vi "Error.vi"(6 "Station":T1(ring), 7 "timeout ms (-1)":i32=-1, 8 "error out":errorcluster, 9 "VI Name":string, 10 "error":errorcluster, 11 "Socket":i32) -> (0 "error out 2":errorcluster)   [LabVIEW 2019, in "Unit Test Engine Tools.lvlib"]
uses:
  Unit Test Engine Tools.lvlib
  LVUT Global 1.vi
  <resource>/objmgr/ni.dex.rc
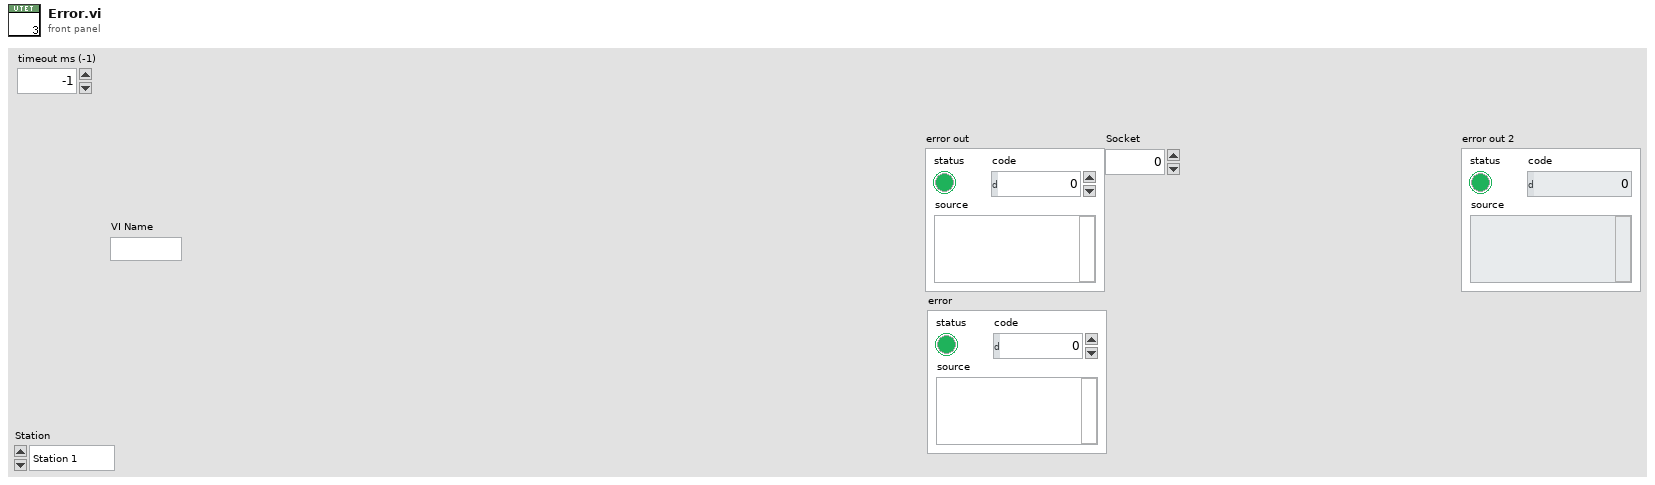
[diagram p1: front panel]
types:
  T1 = enum16{"Station 1", "Station 2", "Station 3", "Station 4"}
  T2 = cluster{"Socket":i32, "error in":errorcluster, "VI Name":string}
  T3 = cluster{"Socket":i32, "error IO":errorcluster, "VI Name":string}
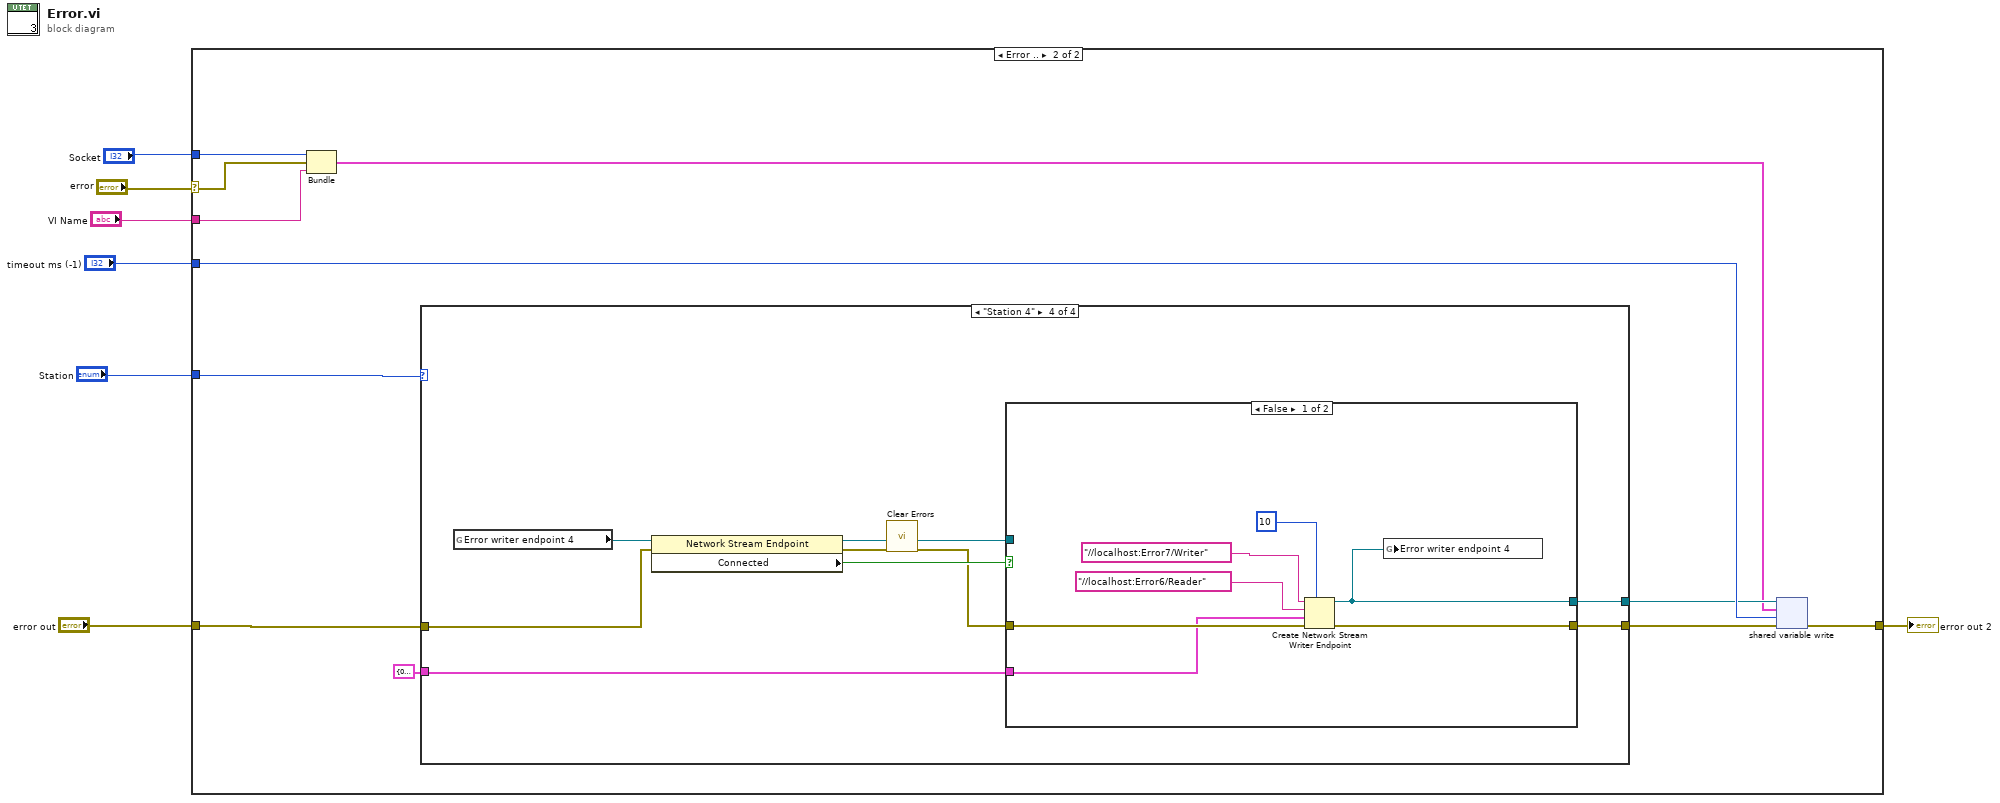
[diagram p0: block diagram]
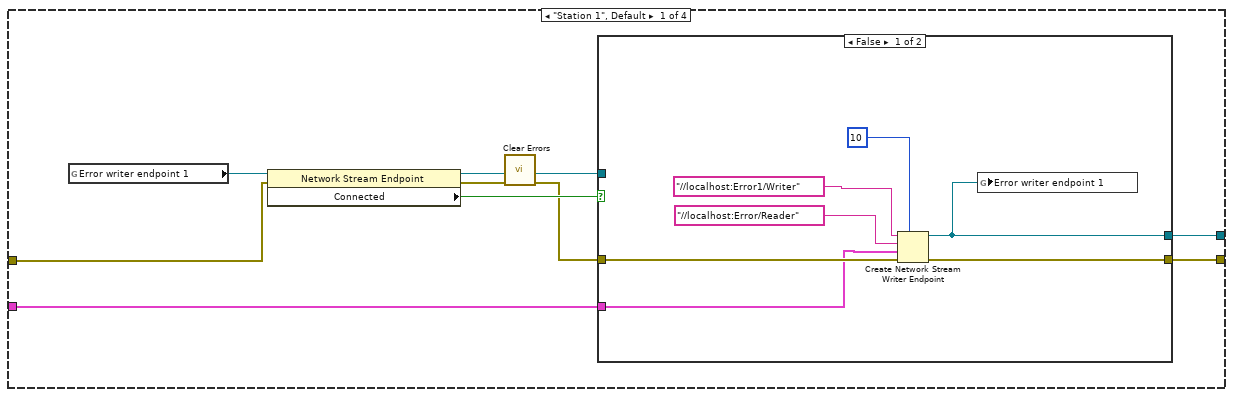
[diagram p3: hidden frame]
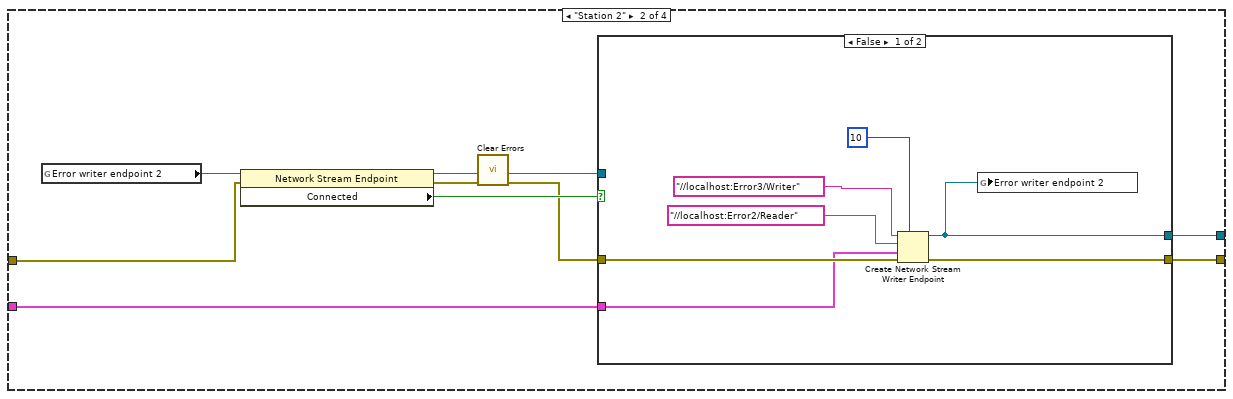
[diagram p5: hidden frame]
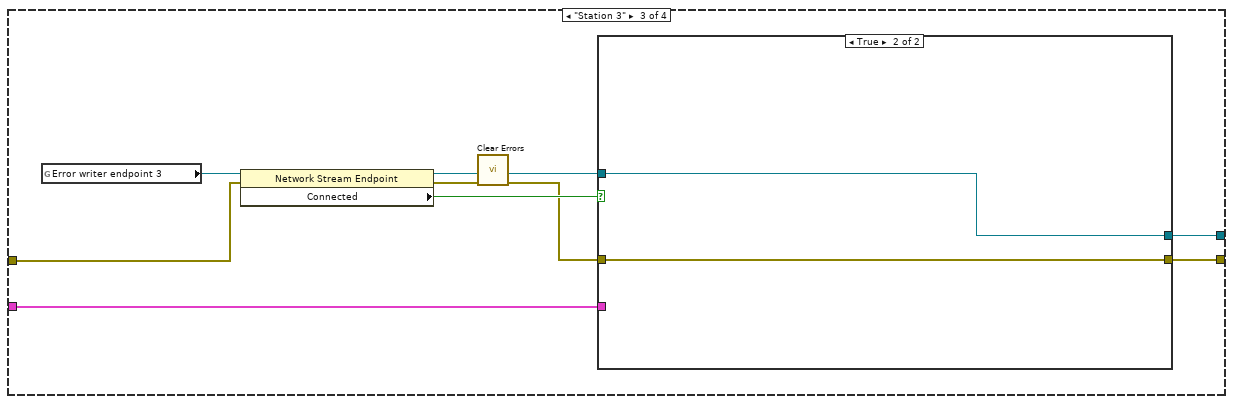
[diagram p7: hidden frame]
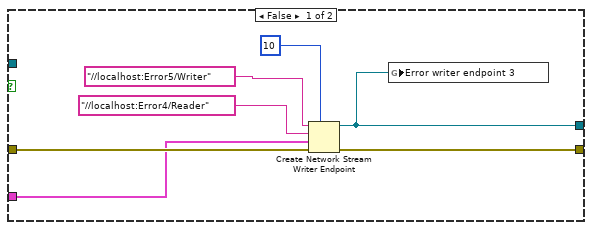
[diagram p8: hidden frame]
diagram:
  n1 = case shown="Error .." "error" {
    selector: "error" -> [_ w11]
    tunnel: "Station" -> [_ w19]
    tunnel: "timeout ms (-1)" -> [_ w18]
    tunnel: "error out" -> [w8 w15]
    tunnel: [w8 w14] -> w4
    tunnel: "Socket" -> [_ w12]
    tunnel: "VI Name" -> [_ w9]
    frame No Error {
    }
    frame Error {
      n2 = Bundle("Socket"=w12, "error IO"=w11, "VI Name"=w9) -> (w10:T3)  [unwired: 1 in]
      n3 = case shown="\"Station 4\"" w19 {
        tunnel: [w22 w40 w58 w75] -> w17
        tunnel: w15 -> [w24 w42 w60 w78]
        tunnel: [w21 w39 w57 w76] -> w16
        tunnel: T2 {"Socket"=0, "error in"={"status"=FALSE, "code"=0, "source"=""}, "VI Name"=""} -> [w20 w38 w56 w74]
        frame "Station 1", Default {
          n4 = global read "LVUT Global 1.vi" "Error writer endpoint 1"() -> (w28:refnum<k21>)
          n5 = property class="Network Stream Endpoint"(reference=w28, error in=w24) -> (reference out=w25:refnum<k21>, error out=w27:errorcluster, "Connected"=w26:bool)
          n6 = call <vilib>:"Clear Errors.vi"("error in (no error)"=w27) -> ("error out"=w23:errorcluster)  [unwired: 5 in, 1 out]
          n7 = case shown="False" w26 {
            tunnel: [w29 w37] -> w21
            tunnel: [w34 w36] -> w22
            tunnel: w23 -> [w31 w36]
            tunnel: w25 -> [_ w37]
            tunnel: w20 -> [w30 _]
            frame False {
              n8 = Create Network Stream Writer Endpoint(7:10 ("writer buffer size"), 8:w31, 9:w30, 10:"//localhost:Error/Reader" ("reader name"), 11:"//localhost:Error1/Writer" ("reader name")) -> (0:w34:errorcluster, 3:w29:refnum<k21>)  [unwired: 2 in]
              n9 = global write "LVUT Global 1.vi" "Error writer endpoint 1"(w29) -> ()
            }
            frame True {
            }
          }
        }
        frame "Station 2" {
          n10 = global read "LVUT Global 1.vi" "Error writer endpoint 2"() -> (w46:refnum<k21>)
          n11 = property class="Network Stream Endpoint"(reference=w46, error in=w42) -> (reference out=w43:refnum<k21>, error out=w45:errorcluster, "Connected"=w44:bool)
          n12 = call <vilib>:"Clear Errors.vi"("error in (no error)"=w45) -> ("error out"=w41:errorcluster)  [unwired: 5 in, 1 out]
          n13 = case shown="False" w44 {
            tunnel: [w48 w55] -> w39
            tunnel: [w52 w54] -> w40
            tunnel: w41 -> [w49 w54]
            tunnel: w43 -> [_ w55]
            tunnel: w38 -> [w47 _]
            frame False {
              n14 = Create Network Stream Writer Endpoint(7:10 ("writer buffer size"), 8:w49, 9:w47, 10:"//localhost:Error2/Reader" ("reader name"), 11:"//localhost:Error3/Writer" ("reader name")) -> (0:w52:errorcluster, 3:w48:refnum<k21>)  [unwired: 2 in]
              n15 = global write "LVUT Global 1.vi" "Error writer endpoint 2"(w48) -> ()
            }
            frame True {
            }
          }
        }
        frame "Station 3" {
          n16 = global read "LVUT Global 1.vi" "Error writer endpoint 3"() -> (w64:refnum<k21>)
          n17 = property class="Network Stream Endpoint"(reference=w64, error in=w60) -> (reference out=w61:refnum<k21>, error out=w63:errorcluster, "Connected"=w62:bool)
          n18 = call <vilib>:"Clear Errors.vi"("error in (no error)"=w63) -> ("error out"=w59:errorcluster)  [unwired: 5 in, 1 out]
          n19 = case shown="True" w62 {
            tunnel: [w66 w73] -> w57
            tunnel: [w70 w72] -> w58
            tunnel: w59 -> [w67 w72]
            tunnel: w61 -> [_ w73]
            tunnel: w56 -> [w65 _]
            frame False {
              n20 = Create Network Stream Writer Endpoint(7:10 ("writer buffer size"), 8:w67, 9:w65, 10:"//localhost:Error4/Reader" ("reader name"), 11:"//localhost:Error5/Writer" ("reader name")) -> (0:w70:errorcluster, 3:w66:refnum<k21>)  [unwired: 2 in]
              n21 = global write "LVUT Global 1.vi" "Error writer endpoint 3"(w66) -> ()
            }
            frame True {
            }
          }
        }
        frame "Station 4" {
          n22 = global read "LVUT Global 1.vi" "Error writer endpoint 4"() -> (w82:refnum<k21>)
          n23 = property class="Network Stream Endpoint"(reference=w82, error in=w78) -> (reference out=w79:refnum<k21>, error out=w81:errorcluster, "Connected"=w80:bool)
          n24 = call <vilib>:"Clear Errors.vi"("error in (no error)"=w81) -> ("error out"=w77:errorcluster)  [unwired: 5 in, 1 out]
          n25 = case shown="False" w80 {
            tunnel: [w84 w91] -> w76
            tunnel: [w88 w90] -> w75
            tunnel: w77 -> [w85 w90]
            tunnel: w79 -> [_ w91]
            tunnel: w74 -> [w83 _]
            frame False {
              n26 = Create Network Stream Writer Endpoint(7:10 ("writer buffer size"), 8:w85, 9:w83, 10:"//localhost:Error6/Reader" ("reader name"), 11:"//localhost:Error7/Writer" ("reader name")) -> (0:w88:errorcluster, 3:w84:refnum<k21>)  [unwired: 2 in]
              n27 = global write "LVUT Global 1.vi" "Error writer endpoint 4"(w84) -> ()
            }
            frame True {
            }
          }
        }
      }
      n28 = shared-variable-write(w16, w17, w10, w18) -> (w14:errorcluster)  [unwired: 2 out]
    }
  }
  "error out 2" <- w4
